vi "Prog Interface - TREE.vi"() -> ()   [LabVIEW 2017, in "Nanonis Prog Interface.lvlib"]
uses:
  Nanonis Prog Interface.lvlib
  <userlib>/Nanonis Prog Interface V5/Scan/Piezos/Piezo Calibration Sens Set.vi
  <userlib>/Nanonis Prog Interface V5/Scan/Piezos/Piezo Calibration Sens Get.vi
  <userlib>/Nanonis Prog Interface V5/Scan/Grid/GridPatternSet.vi
  <userlib>/Nanonis Prog Interface V5/Scan/Grid/GridPatternGet.vi
panel:
  in  "Tab Control":enum32{"Readme", "Version history"}(tab)=enum."Version history"
  in  "Version history":string="*** R8177 (September 2018) ***\n\nNew functions to get/set the limits of the User Outputs.\nNew functions to get values from the measurements list.\nAdapted function to get/set the properties of the Lockin Frequency Sweep.\n\n-----------------------------------------------------------------------------------------------------\n\n*** R8101 (September 2018) ***\n\nAdapted function to set the Idle value of the Fast Output from any connected SC5.\nAdapted function to get parameters from all modules to retrieve also the parameters grouped by module.\nAdapted function to get/set Scan properties to include the modules parameters selected in the Scan Control.\nNew function to open the Data Logger module.\nNew functions to get/set the XYZ voltage limits in the Piezo Calibration module.\nAdded option to wait until the tip stops withdrawing in the Withdraw function.\n\n-----------------------------------------------------------------------------------------------------\n\n*** R7861 (April 2018) ***\n\nNew functions palette for the Data Logger module.\n\n-----------------------------------------------------------------------------------------------------\n\n*** R7824 (April 2018) ***\n\nAdapted functions to the get/set the 2nd Auto Retract condition in the Z-Spectroscopy module.\n\n-----------------------------------------------------------------------------------------------------\n\n*** R7703 (February 2018) ***\n\nAdapted functions to the new number of available Real Time signals in the Nanonis software. \nThe full list of signals has increased from 80 to 128.\n\nAdded settling time to get/set properties of the Generic sweeper.\nAdded new functions to get/set Bias Spectroscopy options in the Advanced section.\nAdded optimizations to the get/set pattern functions when doing experiments on a grid.\n\n-----------------------------------------------------------------------------------------------------\n\n*** R7296 (June 2017) ***\n\nAdded functions to load/save LUTs in the Script-LUT Editor.\nIncreased the maximum number of steps allowed in the Generic Sweeper.\nAdded example to convert black pixels of an image into scan coordinates.\n\n-----------------------------------------------------------------------------------------------------\n\n*** R6949 (November 2016) ***\n\nAdded functions to get/set the configuration options in the Oscilation Control Signal Analyzer and Zoom FFT modules.\nDocumentation fix for Generic PI Controller.\n\n-----------------------------------------------------------------------------------------------------\n\n*** R6864 (October 2016) ***\n\nAdded a new function to set the Session folder.\n\n-----------------------------------------------------------------------------------------------------\n\n*** R6828 (September 2016) ***\n\nAdded new functions for the Function Generator (2 Channels) module.\nAdded new functions to Get / Set name and SI units of USer Outputs and User Inputs.\nAdded some VIs to the \"TREE.vi\" which were previously missing.\n\n-----------------------------------------------------------------------------------------------------\n\n*** R6778 (August 2016) ***\n\nAdded new functions for Modulator and demodulator channel set and get for Lockin, moved old VIs to Legacy (Removed from palettes).\nAdded Generic PI functions to set input and output channels.\n\n-----------------------------------------------------------------------------------------------------\n\n*** R6727 (August 2016) ***\n\nAdaptation to software with 80 channels and support for up to 3 SC5s, providing up to 16 additional outputs and 16 additional input channels.\n\n-----------------------------------------------------------------------------------------------------\n\n*** R6313 (March 2016) ***\n\nAdded Modulator phase offset to Lockin API\n\n-----------------------------------------------------------------------------------------------------\n\n*** R6310 (February 2016) ***\n\nNew functions to control the new Lock-in module. The old functions are still available as legacy VIs, but we strongly recommend using the new function set.\nNew functions for the Script module.\nNew example: History Chart 1-Channel (similar to the software built-in History graph)\n\n-----------------------------------------------------------------------------------------------------\n\n*** R6213 (January 2016) ***\n\nSome functions fixed.\n\n-----------------------------------------------------------------------------------------------------\n\n*** R6104 (November 2015) ***\n\nNew functions to load/save layouts, and to show/hide the PSD section of the High Resolution Oscilloscope.\n\n-----------------------------------------------------------------------------------------------------\n\n*** R5929 (October 2015) ***\n\nNew functions to draw multiple points and lines in the scan display.\n\n-----------------------------------------------------------------------------------------------------\n\n*** R5882 (September 2015) ***\n\nNew functions to get/set the Trigger Level value in the Oscilloscope High Resolution graph.\n\n-----------------------------------------------------------------------------------------------------\n\n*** R5864 (September 2015) ***\n\nNew functions to get/set the Withdraw Slew Rate in Z-Controller.\n\n-----------------------------------------------------------------------------------------------------\n\n*** R5786 (August 2015) ***\n\nNew functions to load/save settings files.\n\n-----------------------------------------------------------------------------------------------------\n\n*** R5706 (July 2015) ***\n\nThe examples are no longer part of the Nanonis library.\n\n-----------------------------------------------------------------------------------------------------\n\n*** R5681 (July 2015) ***\n\nNew function to open the Oscilloscope High Resolution graph.\n\n-----------------------------------------------------------------------------------------------------\n\n*** R5638 (June 2015) ***\n\nNew functions to control the Oscilloscope High Resolution graph.\nNew arrangement of functions inside subpalettes  in the Graphs palette.\nAdded more properties to the Properties Get/Set functions for Bias and Z spectroscopies.\n\n-----------------------------------------------------------------------------------------------------\n\n\n*** R5526 (April 2015) ***\n\nNew function to determine the optimal PLL gains.\n\n-----------------------------------------------------------------------------------------------------\n\n*** R5443 (March 2015) ***\n\nMultipass Callback VI example added a new input called \"Method\" to the connector pane. Now the Multipass example allows to execute user-defined code before (\"init\"), during (\"run\"), and after (\"end\") the scan.\n\n-----------------------------------------------------------------------------------------------------\n\n*** R5350 (February 2015) ***\n\nNew VIs in the Z-Controller palette to enable, get and set the Z limits.\n\n-----------------------------------------------------------------------------------------------------\n\n*** V5 first release R5286 (February 2015) ***\n\n-----------------------------------------------------------------------------------------------------\n\n*** R4760 (September 2014) ***\n\nNew VIs in the Current palette to get and set the calibration and offset.\n\n-----------------------------------------------------------------------------------------------------\n\n*** R4695 (June 2014) ***\n\nNew VIs in the Generic Sweeper palette to get properties and limits, and to stop the sweep.\n\n-----------------------------------------------------------------------------------------------------\n\n*** R4647 (May 2014) ***\n\nNew VIs to access the Global Counter.\n\n-----------------------------------------------------------------------------------------------------\n\n*** R4602 (April 2014) ***\n\nChanged VI:\n- HVA Info Get: added AUX gain.\n\n\n-----------------------------------------------------------------------------------------------------\n\n*** R4540 (February 2014) ***\n\nNew VIs:\n- Oscillation Control /-2 Lock-in Harmonic get / set\n- PLL Signal Analyzer and ZoomFFT: Open module, Channels get / set\n\nChanged VI:\n- Scan Speed Get / Set: added Bwd-Fwd Speed Ratio.\n\n\n-----------------------------------------------------------------------------------------------------\n\n*** R4316 (November 2013) ***\nNanonis Programming Interface V4.5 built by the VI Package Manager for the first time\n\n\n-----------------------------------------------------------------------------------------------------\n\n*** R4234 (October 2013) ***\n- New VIs to get/set the Beam Deflection configuration, in the Laser palette\n- New VIs to get/set the signals configuration in the Signals Manager, in the Signals palette\n\n\n-----------------------------------------------------------------------------------------------------\n\n*** V4.5 first release R3807 (May 2013) ***\nBased on Programming Interface V4.0, but including some changes:\n- Signal VIs adapted to the 48 signals available in V4.5\n- Support for new V4.5 Lock-in (FPGA Lock-in) and Oscilloscope 2T\n- New VIs to get/set the Function Generator idle value\n- Some other changes due to V4.5 modifications in the software"
  # "Programming Interface V5"
  # "See block diagram for VI TREE"
  # "1) What is the Programming Interface?\n\nThe Programming Interface is a set of LabVIEW VIs to control many functions of the Nanonis Controller Software.\n\n2) Location\n\nThe files are installed by default in the \"user.lib\" folder of LabVIEW.\nThus, the Programming Interface VIs are directly available from the LabVIEW function palette under the \"User libraries\" section. \nThe \"TREE.vi\" VI is not meant to be run but to display all the available VIs. \n\n3) Remote access\n\nIf you want to use the Programming Interface from another PC than the one on which the Nanonis Controller Software is running, you first have to enable the access from the Nanonis Software. \nTo do so, from the Nanonis Software main window, open the \"System>Options\" window and nagivate to \"Programming Interface\".\nIn the \"Machine access configuration\", add the IP address of the PC on which the Programming Interface VIs are running.\nMake sure your software firewall allows access from the remote PC. Depending on your software firewall you can add the remote PC in trusted environment or you can allow \"Nanonis SPM Controller.exe\" to listen to incoming connections and add port 3364 to the exceptions list.\n\n4) Examples\n\nSeveral example VIs are located in the \"Nanonis Prog Interface/Examples\" palette section."
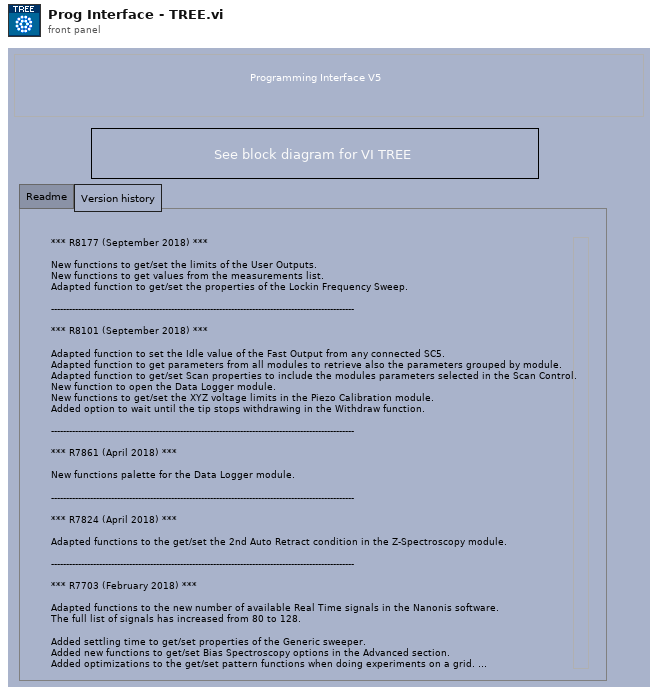
[diagram p1: front panel]
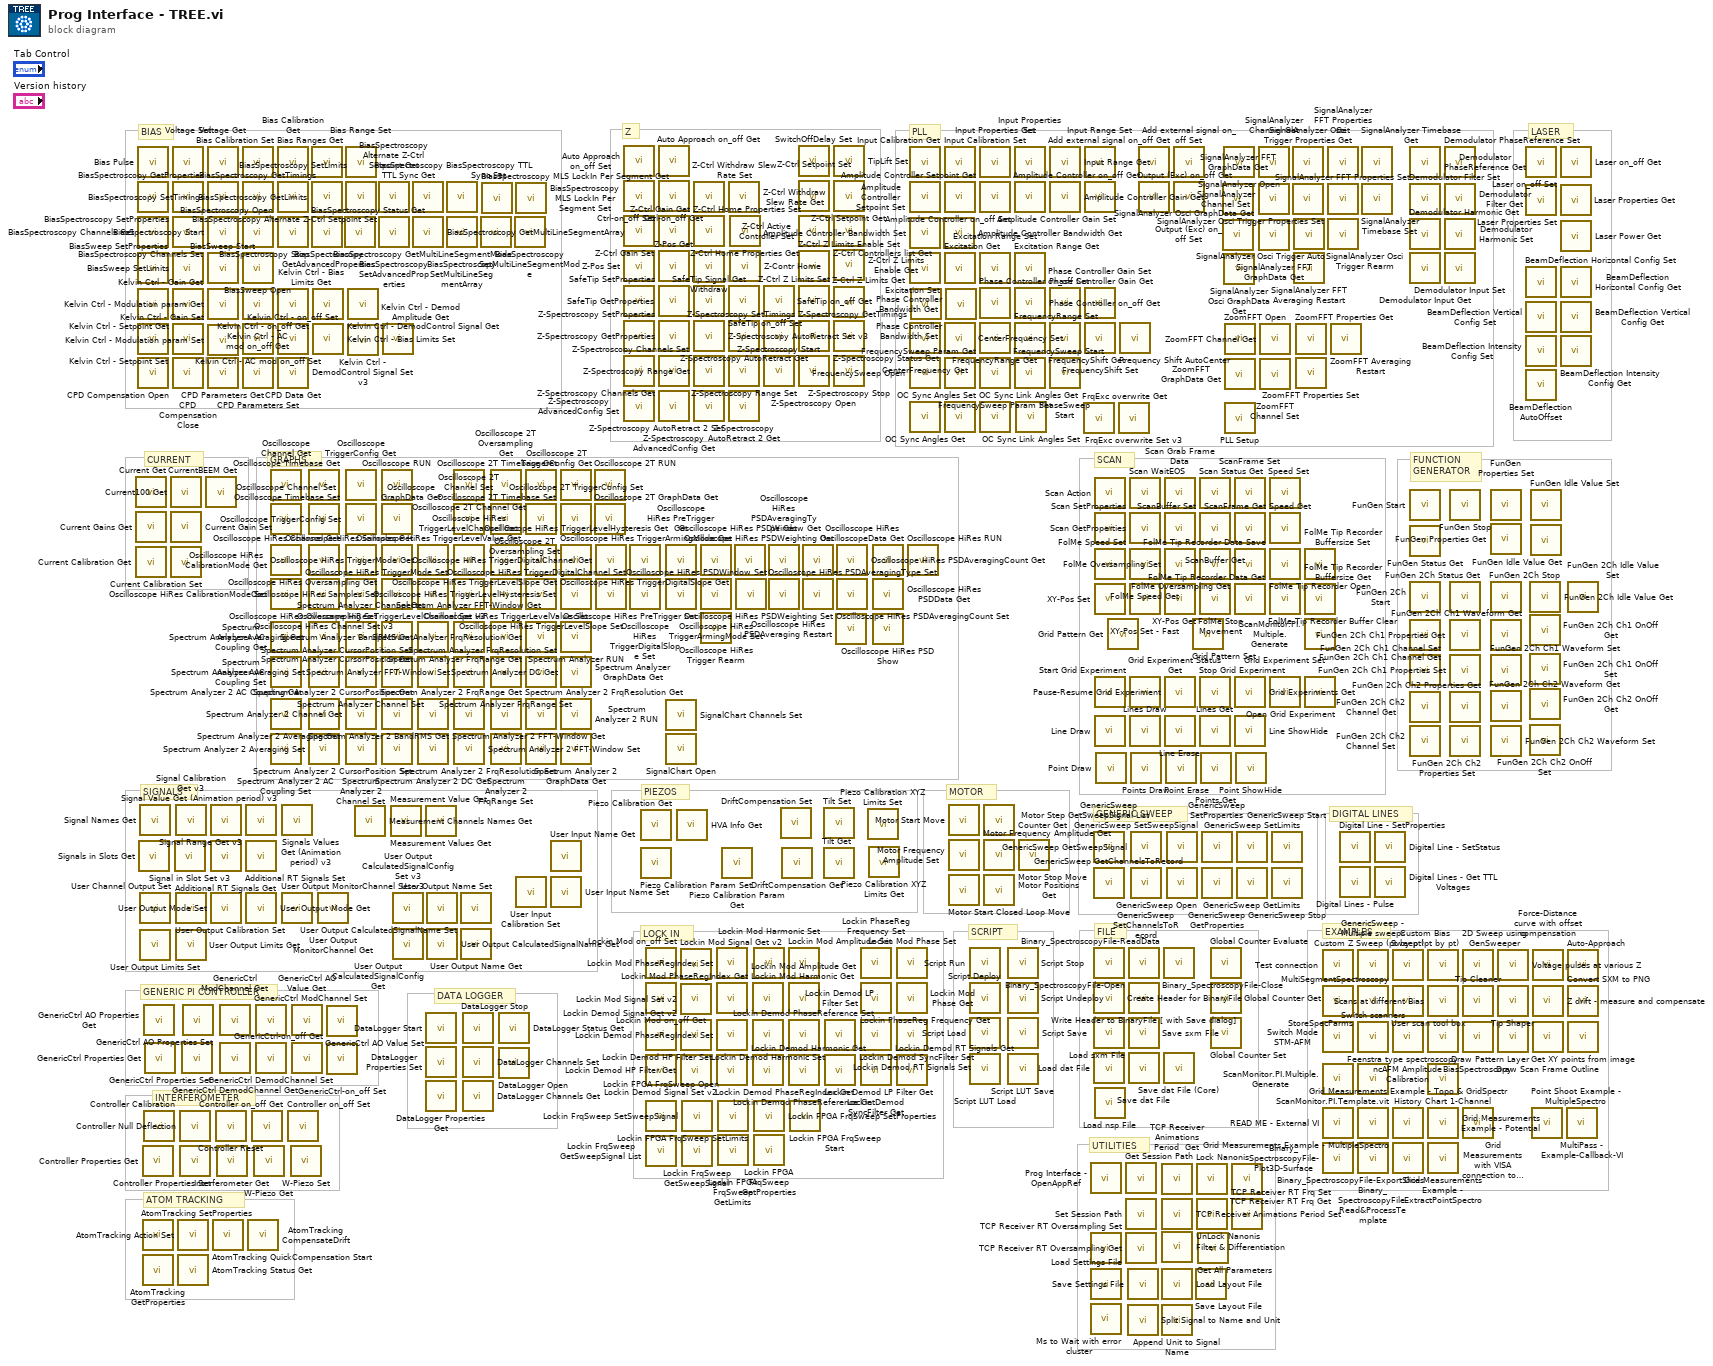
[diagram p0: block diagram]
diagram:
  # "DATA LOGGER"
  # "SCRIPT"
  # "LOCK IN"
  # "FUNCTION\nGENERATOR"
  # "GENERIC PI CONTROLLER"
  # "INTERFEROMETER"
  # "GRAPHS"
  # "LASER"
  # "ATOM TRACKING"
  # "PIEZOS"
  # "DIGITAL LINES"
  # "FILE"
  # "Z"
  # "UTILITIES"
  # "GENERIC SWEEP"
  # "SIGNALS"
  # "SCAN"
  # "PLL"
  # "EXAMPLES"
  # "CURRENT"
  # "MOTOR"
  # "BIAS"
  n1 = call <userlib>:"Current Get.vi"() -> ()  [unwired: 7 in, 3 out]
  n2 = call <userlib>:"Current Gains Get.vi"() -> ()  [unwired: 8 in, 4 out]
  n3 = call <userlib>:"Current Calibration Get.vi"() -> ()  [unwired: 8 in, 4 out]
  n4 = call <userlib>:"Bias Pulse.vi"() -> ()  [unwired: 14 in, 2 out]
  n5 = call <userlib>:"BiasSpectroscopy SetProperties.vi"() -> ()  [unwired: 14 in, 2 out]
  n6 = call <userlib>:"BiasSpectroscopy Channels Get.vi"() -> ()  [unwired: 9 in, 3 out]
  n7 = call <userlib>:"BiasSweep SetProperties.vi"() -> ()  [unwired: 14 in, 2 out]
  n8 = call <userlib>:"Kelvin Ctrl - Setpoint Get.vi"() -> ()  [unwired: 9 in, 3 out]
  n9 = call <userlib>:"Kelvin Ctrl - Setpoint Set.vi"() -> ()  [unwired: 10 in, 2 out]
  n10 = call <userlib>:"CPD Compensation Open.vi"() -> ()  [unwired: 14 in, 2 out]
  n11 = call <userlib>:"Signals in Slots Get.vi"() -> ()  [unwired: 6 in, 4 out]
  n12 = call <instrlib>:"Signal Names Get.vi"() -> ()  [unwired: 7 in, 3 out]
  n13 = call <userlib>:"User Channel Output Set.vi"() -> ()  [unwired: 9 in, 2 out]
  n14 = call <userlib>:"User Output Limits Set.vi"() -> ()  [unwired: 14 in, 2 out]
  n15 = call <userlib>:"Controller Properties Get.vi"() -> ()  [unwired: 11 in, 5 out]
  n16 = call <userlib>:"AtomTracking SetProperties.vi"() -> ()  [unwired: 14 in, 2 out]
  n17 = call <userlib>:"AtomTracking GetProperties.vi"() -> ()  [unwired: 9 in, 7 out]
  n18 = call <userlib>:"GenericCtrl AO Properties Get.vi"() -> ()  [unwired: 4 in, 8 out]
  n19 = call <userlib>:"Controller Calibration.vi"() -> ()  [unwired: 10 in, 2 out]
  n20 = call <userlib>:"GenericCtrl Properties Get.vi"() -> ()  [unwired: 6 in, 6 out]
  n21 = call <userlib>:"Current100 Get.vi"() -> ()  [unwired: 7 in, 3 out]
  n22 = call <userlib>:"Current Gain Set.vi"() -> ()  [unwired: 10 in, 2 out]
  n23 = call <userlib>:"Current Calibration Set.vi"() -> ()  [unwired: 10 in, 2 out]
  n24 = call <userlib>:"Voltage Set.vi"() -> ()  [unwired: 10 in, 2 out]
  n25 = call <userlib>:"BiasSpectroscopy GetProperties.vi"() -> ()  [unwired: 8 in, 8 out]
  n26 = call <userlib>:"BiasSpectroscopy Channels Set.vi"() -> ()  [unwired: 10 in, 2 out]
  n27 = call <userlib>:"BiasSweep SetLimits.vi"() -> ()  [unwired: 8 in, 2 out]
  n28 = call <userlib>:"Kelvin Ctrl - Gain Get.vi"() -> ()  [unwired: 11 in, 5 out]
  n29 = call <userlib>:"Kelvin Ctrl - Gain Set.vi"() -> ()  [unwired: 14 in, 2 out]
  n30 = call <userlib>:"CPD Compensation Close.vi"() -> ()  [unwired: 14 in, 2 out]
  n31 = call <userlib>:"Signal in Slot Set v3.vi"() -> ()  [unwired: 8 in, 2 out]
  n32 = call <userlib>:"Signal Calibration Get v3.vi"() -> ()  [unwired: 7 in, 4 out]
  n33 = call <userlib>:"User Output Calibration Set.vi"() -> ()  [unwired: 14 in, 2 out]
  n34 = call <userlib>:"User Output Limits Get.vi"() -> ()  [unwired: 12 in, 4 out]
  n35 = call <userlib>:"AtomTracking Action Set.vi"() -> ()  [unwired: 10 in, 2 out]
  n36 = call <userlib>:"AtomTracking Status Get.vi"() -> ()  [unwired: 9 in, 3 out]
  n37 = call <userlib>:"Controller Null Deflection.vi"() -> ()  [unwired: 10 in, 2 out]
  n38 = call <userlib>:"Controller Properties Set.vi"() -> ()  [unwired: 14 in, 2 out]
  n39 = call <userlib>:"GenericCtrl Properties Set.vi"() -> ()  [unwired: 10 in, 2 out]
  n40 = call <userlib>:"GenericCtrl AO Properties Set.vi"() -> ()  [unwired: 10 in, 2 out]
  n41 = call <userlib>:"CurrentBEEM Get.vi"() -> ()  [unwired: 7 in, 3 out]
  n42 = call <userlib>:"Voltage Get.vi"() -> ()  [unwired: 9 in, 3 out]
  n43 = call <userlib>:"BiasSpectroscopy SetTimings.vi"() -> ()  [unwired: 14 in, 2 out]
  n44 = call <userlib>:"BiasSpectroscopy Start.vi"() -> ()  [unwired: 11 in, 5 out]
  n45 = call <userlib>:"BiasSweep Start.vi"() -> ()  [unwired: 8 in, 4 out]
  n46 = call <userlib>:"Kelvin Ctrl - Modulation param Get.vi"() -> ()  [unwired: 11 in, 5 out]
  n47 = call <userlib>:"Kelvin Ctrl - Modulation param Set.vi"() -> ()  [unwired: 14 in, 2 out]
  n48 = call <userlib>:"CPD Parameters Get.vi"() -> ()  [unwired: 11 in, 5 out]
  n49 = call <userlib>:"Signal Range Get v3.vi"() -> ()  [unwired: 7 in, 4 out]
  n50 = call <userlib>:"Additional RT Signals Get.vi"() -> ()  [unwired: 11 in, 5 out]
  n51 = call <userlib>:"User Output Mode Set.vi"() -> ()  [unwired: 9 in, 2 out]
  n52 = call <userlib>:"AtomTracking QuickCompensation Start.vi"() -> ()  [unwired: 10 in, 2 out]
  n53 = call <userlib>:"Controller Reset.vi"() -> ()  [unwired: 10 in, 2 out]
  n54 = call <userlib>:"Interferometer Get.vi"() -> ()  [unwired: 9 in, 3 out]
  n55 = call <userlib>:"GenericCtrl ModChannel Get.vi"() -> ()  [unwired: 9 in, 3 out]
  n56 = call <userlib>:"GenericCtrl DemodChannel Get.vi"() -> ()  [unwired: 9 in, 3 out]
  n57 = call <userlib>:"Bias Calibration Set.vi"() -> ()  [unwired: 10 in, 2 out]
  n58 = call <userlib>:"BiasSpectroscopy GetTimings.vi"() -> ()  [unwired: 11 in, 5 out]
  n59 = call <userlib>:"BiasSpectroscopy Open.vi"() -> ()  [unwired: 14 in, 2 out]
  n60 = call <userlib>:"BiasSweep Open.vi"() -> ()  [unwired: 14 in, 2 out]
  n61 = call <userlib>:"Kelvin Ctrl - AC mod on_off Get.vi"() -> ()  [unwired: 8 in, 4 out]
  n62 = call <userlib>:"Kelvin Ctrl - AC mod on_off Set.vi"() -> ()  [unwired: 10 in, 2 out]
  n63 = call <userlib>:"CPD Parameters Set.vi"() -> ()  [unwired: 14 in, 2 out]
  n64 = call <instrlib>:"Signal Value Get (Animation period) v3.vi"() -> ()  [unwired: 8 in, 3 out]
  n65 = call <userlib>:"Additional RT Signals Set.vi"() -> ()  [unwired: 8 in, 2 out]
  n66 = call <userlib>:"User Output Mode Get.vi"() -> ()  [unwired: 7 in, 3 out]
  n67 = call <userlib>:"AtomTracking CompensateDrift.vi"() -> ()  [unwired: 10 in, 2 out]
  n68 = call <userlib>:"Controller on_off Get.vi"() -> ()  [unwired: 9 in, 3 out]
  n69 = call <userlib>:"W-Piezo Get.vi"() -> ()  [unwired: 9 in, 3 out]
  n70 = call <userlib>:"GenericCtrl ModChannel Set.vi"() -> ()  [unwired: 10 in, 2 out]
  n71 = call <userlib>:"GenericCtrl DemodChannel Set.vi"() -> ()  [unwired: 10 in, 2 out]
  n72 = call <userlib>:"Oscilloscope Channel Get.vi"() -> ()  [unwired: 9 in, 3 out]
  n73 = call <userlib>:"Oscilloscope Channel Set.vi"() -> ()  [unwired: 10 in, 2 out]
  n74 = call <userlib>:"Oscilloscope HiRes CalibrationMode Get.vi"() -> ()  [unwired: 9 in, 3 out]
  n75 = call <userlib>:"Oscilloscope HiRes CalibrationMode Set.vi"() -> ()  [unwired: 10 in, 2 out]
  n76 = call <userlib>:"Spectrum Analyzer AC Coupling Get.vi"() -> ()  [unwired: 9 in, 3 out]
  n77 = call <userlib>:"Spectrum Analyzer AC Coupling Set.vi"() -> ()  [unwired: 10 in, 2 out]
  n78 = call <userlib>:"Spectrum Analyzer 2 AC Coupling Get.vi"() -> ()  [unwired: 9 in, 3 out]
  n79 = call <userlib>:"Spectrum Analyzer 2 AC Coupling Set.vi"() -> ()  [unwired: 10 in, 2 out]
  n80 = call <userlib>:"Bias Calibration Get.vi"() -> ()  [unwired: 8 in, 4 out]
  n81 = call <userlib>:"BiasSpectroscopy SetLimits.vi"() -> ()  [unwired: 8 in, 2 out]
  n82 = call <userlib>:"BiasSpectroscopy Stop.vi"() -> ()  [unwired: 14 in, 2 out]
  n83 = call <userlib>:"Kelvin Ctrl - on_off Get.vi"() -> ()  [unwired: 9 in, 3 out]
  n84 = call <userlib>:"Kelvin Ctrl - on_off Set.vi"() -> ()  [unwired: 10 in, 2 out]
  n85 = call <userlib>:"CPD Data Get.vi"() -> ()  [unwired: 11 in, 5 out]
  n86 = call <userlib>:"Signals Values Get (Animation period) v3.vi"() -> ()  [unwired: 8 in, 3 out]
  n87 = call <userlib>:"User Output MonitorChannel Set v3.vi"() -> ()  [unwired: 9 in, 2 out]
  n88 = call <userlib>:"Controller on_off Set.vi"() -> ()  [unwired: 10 in, 2 out]
  n89 = call <userlib>:"W-Piezo Set.vi"() -> ()  [unwired: 10 in, 2 out]
  n90 = call <userlib>:"GenericCtrl AO Value Get.vi"() -> ()  [unwired: 9 in, 3 out]
  n91 = call <userlib>:"GenericCtrl-on_off Get.vi"() -> ()  [unwired: 9 in, 3 out]
  n92 = call <userlib>:"Oscilloscope Timebase Get.vi"() -> ()  [unwired: 8 in, 4 out]
  n93 = call <userlib>:"Oscilloscope Timebase Set.vi"() -> ()  [unwired: 10 in, 2 out]
  n94 = call <userlib>:"Oscilloscope HiRes Channel Get.vi"() -> ()  [unwired: 9 in, 3 out]
  n95 = call <userlib>:"Oscilloscope HiRes Channel Set v3.vi"() -> ()  [unwired: 10 in, 2 out]
  n96 = call <userlib>:"Spectrum Analyzer Averaging Get.vi"() -> ()  [unwired: 9 in, 3 out]
  n97 = call <userlib>:"Spectrum Analyzer Averaging Set.vi"() -> ()  [unwired: 10 in, 2 out]
  n98 = call <userlib>:"Spectrum Analyzer 2 Averaging Get.vi"() -> ()  [unwired: 9 in, 3 out]
  n99 = call <userlib>:"Spectrum Analyzer 2 Averaging Set.vi"() -> ()  [unwired: 10 in, 2 out]
  n100 = call <userlib>:"Bias Ranges Get.vi"() -> ()  [unwired: 8 in, 4 out]
  n101 = call <userlib>:"BiasSpectroscopy GetLimits.vi"() -> ()  [unwired: 6 in, 4 out]
  n102 = call <userlib>:"BiasSpectroscopy Status Get.vi"() -> ()  [unwired: 7 in, 3 out]
  n103 = call <userlib>:"Kelvin Ctrl - Bias Limits Get.vi"() -> ()  [unwired: 8 in, 4 out]
  n104 = call <userlib>:"Kelvin Ctrl - Bias Limits Set.vi"() -> ()  [unwired: 10 in, 2 out]
  n105 = call <userlib>:"User Output MonitorChannel Get.vi"() -> ()  [unwired: 8 in, 3 out]
  n106 = call <userlib>:"GenericCtrl AO Value Set.vi"() -> ()  [unwired: 10 in, 2 out]
  n107 = call <userlib>:"GenericCtrl-on_off Set.vi"() -> ()  [unwired: 10 in, 2 out]
  n108 = call <userlib>:"BiasSpectroscopy GetAdvancedProperties.vi"() -> ()  [unwired: 10 in, 6 out]
  n109 = call <userlib>:"Bias Range Set.vi"() -> ()  [unwired: 10 in, 2 out]
  n110 = call <userlib>:"BiasSpectroscopy Alternate Z-Ctrl Setpoint Set.vi"() -> ()  [unwired: 14 in, 2 out]
  n111 = call <userlib>:"Oscilloscope TriggerConfig Get.vi"() -> ()  [unwired: 8 in, 4 out]
  n112 = call <userlib>:"Oscilloscope TriggerConfig Set.vi"() -> ()  [unwired: 10 in, 2 out]
  n113 = call <userlib>:"Oscilloscope HiRes Oversampling Get.vi"() -> ()  [unwired: 9 in, 3 out]
  n114 = call <userlib>:"Oscilloscope HiRes Oversampling Set.vi"() -> ()  [unwired: 10 in, 2 out]
  n115 = call <userlib>:"Spectrum Analyzer Channel Get.vi"() -> ()  [unwired: 9 in, 3 out]
  n116 = call <userlib>:"Spectrum Analyzer Channel Set.vi"() -> ()  [unwired: 10 in, 2 out]
  n117 = call <userlib>:"Spectrum Analyzer 2 Channel Get.vi"() -> ()  [unwired: 9 in, 3 out]
  n118 = call <userlib>:"Spectrum Analyzer 2 Channel Set.vi"() -> ()  [unwired: 10 in, 2 out]
  n119 = call <userlib>:"Kelvin Ctrl - DemodControl Signal Get.vi"() -> ()  [unwired: 9 in, 3 out]
  n120 = call <userlib>:"Kelvin Ctrl - DemodControl Signal Set v3.vi"() -> ()  [unwired: 10 in, 2 out]
  n121 = call <userlib>:"Measurement Channels Names Get.vi"() -> ()  [unwired: 9 in, 3 out]
  n122 = call <userlib>:"BiasSpectroscopy Alternate Z-Ctrl Setpoint Get.vi"() -> ()  [unwired: 11 in, 5 out]
  n123 = call <userlib>:"BiasSpectroscopy SetAdvancedProperties.vi"() -> ()  [unwired: 14 in, 2 out]
  n124 = call <userlib>:"Oscilloscope RUN.vi"() -> ()  [unwired: 10 in, 2 out]
  n125 = call <userlib>:"Oscilloscope GraphData Get.vi"() -> ()  [unwired: 9 in, 3 out]
  n126 = call <userlib>:"Oscilloscope HiRes Samples Get.vi"() -> ()  [unwired: 9 in, 3 out]
  n127 = call <userlib>:"Oscilloscope HiRes Samples Set.vi"() -> ()  [unwired: 10 in, 2 out]
  n128 = call <userlib>:"Spectrum Analyzer CursorPosition Get.vi"() -> ()  [unwired: 11 in, 5 out]
  n129 = call <userlib>:"Spectrum Analyzer CursorPosition Set.vi"() -> ()  [unwired: 14 in, 2 out]
  n130 = call <userlib>:"Spectrum Analyzer 2 CursorPosition Get.vi"() -> ()  [unwired: 11 in, 5 out]
  n131 = call <userlib>:"Spectrum Analyzer 2 CursorPosition Set.vi"() -> ()  [unwired: 14 in, 2 out]
  n132 = call <userlib>:"Kelvin Ctrl - Demod Amplitude Get.vi"() -> ()  [unwired: 9 in, 3 out]
  n133 = call <userlib>:"Measurement Value Get.vi"() -> ()  [unwired: 8 in, 3 out]
  n134 = call <userlib>:"User Output CalculatedSignalConfig Set v3.vi"() -> ()  [unwired: 9 in, 2 out]
  n135 = call <userlib>:"User Output CalculatedSignalConfig Get.vi"() -> ()  [unwired: 8 in, 3 out]
  n136 = call <userlib>:"BiasSpectroscopy TTL Sync Get.vi"() -> ()  [unwired: 9 in, 7 out]
  n137 = call <userlib>:"BiasSpectroscopy GetMultiLineSegmentArray.vi"() -> ()  [unwired: 7 in, 3 out]
  n138 = call <userlib>:"Oscilloscope HiRes TriggerMode Get.vi"() -> ()  [unwired: 9 in, 3 out]
  n139 = call <userlib>:"Oscilloscope HiRes TriggerMode Set.vi"() -> ()  [unwired: 10 in, 2 out]
  n140 = call <userlib>:"Spectrum Analyzer BandRMS Get.vi"() -> ()  [unwired: 8 in, 4 out]
  n141 = call <userlib>:"Spectrum Analyzer DC Get.vi"() -> ()  [unwired: 9 in, 3 out]
  n142 = call <userlib>:"Spectrum Analyzer 2 BandRMS Get.vi"() -> ()  [unwired: 8 in, 4 out]
  n143 = call <userlib>:"Spectrum Analyzer 2 DC Get.vi"() -> ()  [unwired: 9 in, 3 out]
  n144 = call <userlib>:"Measurement Values Get.vi"() -> ()  [unwired: 8 in, 3 out]
  n145 = call <userlib>:"DataLogger Start.vi"() -> ()  [unwired: 14 in, 2 out]
  n146 = call <userlib>:"DataLogger Properties Set.vi"() -> ()  [unwired: 10 in, 2 out]
  n147 = call <userlib>:"DataLogger Properties Get.vi"() -> ()  [unwired: 7 in, 5 out]
  n148 = call <userlib>:"User Output CalculatedSignalName Set.vi"() -> ()  [unwired: 9 in, 2 out]
  n149 = call <userlib>:"User Output CalculatedSignalName Get.vi"() -> ()  [unwired: 8 in, 3 out]
  n150 = call <userlib>:"BiasSpectroscopy TTL Sync Set.vi"() -> ()  [unwired: 14 in, 2 out]
  n151 = call <userlib>:"BiasSpectroscopy SetMultiLineSegmentArray.vi"() -> ()  [unwired: 8 in, 2 out]
  n152 = call <userlib>:"Oscilloscope 2T Channel Get.vi"() -> ()  [unwired: 8 in, 4 out]
  n153 = call <userlib>:"Oscilloscope 2T Channel Set.vi"() -> ()  [unwired: 10 in, 2 out]
  n154 = call <userlib>:"Oscilloscope HiRes TriggerLevelChannel Get.vi"() -> ()  [unwired: 9 in, 3 out]
  n155 = call <userlib>:"Oscilloscope HiRes TriggerLevelChannel Set v3.vi"() -> ()  [unwired: 10 in, 2 out]
  n156 = call <userlib>:"Spectrum Analyzer FFT-Window Get.vi"() -> ()  [unwired: 9 in, 3 out]
  n157 = call <userlib>:"Spectrum Analyzer FFT-Window Set.vi"() -> ()  [unwired: 10 in, 2 out]
  n158 = call <userlib>:"Spectrum Analyzer 2 FFT-Window Get.vi"() -> ()  [unwired: 9 in, 3 out]
  n159 = call <userlib>:"Spectrum Analyzer 2 FFT-Window Set.vi"() -> ()  [unwired: 10 in, 2 out]
  n160 = call <userlib>:"User Output Name Set.vi"() -> ()  [unwired: 14 in, 2 out]
  n161 = call <userlib>:"User Output Name Get.vi"() -> ()  [unwired: 12 in, 4 out]
  n162 = call <userlib>:"DataLogger Stop.vi"() -> ()  [unwired: 14 in, 2 out]
  n163 = call <userlib>:"DataLogger Channels Set.vi"() -> ()  [unwired: 10 in, 2 out]
  n164 = call <userlib>:"DataLogger Channels Get.vi"() -> ()  [unwired: 9 in, 3 out]
  n165 = call <userlib>:"BiasSpectroscopy GetMultiLineSegmentMode.vi"() -> ()  [unwired: 7 in, 3 out]
  n166 = call <userlib>:"BiasSpectroscopy MLS LockIn Per Segment Get.vi"() -> ()  [unwired: 9 in, 3 out]
  n167 = call <userlib>:"Oscilloscope 2T Oversampling Get.vi"() -> ()  [unwired: 8 in, 3 out]
  n168 = call <userlib>:"Oscilloscope 2T Oversampling Set.vi"() -> ()  [unwired: 10 in, 2 out]
  n169 = call <userlib>:"Oscilloscope HiRes TriggerLevelValue Get.vi"() -> ()  [unwired: 9 in, 3 out]
  n170 = call <userlib>:"Oscilloscope HiRes TriggerLevelValue Set.vi"() -> ()  [unwired: 10 in, 2 out]
  n171 = call <userlib>:"Spectrum Analyzer FrqRange Get.vi"() -> ()  [unwired: 8 in, 4 out]
  n172 = call <userlib>:"Spectrum Analyzer FrqRange Set.vi"() -> ()  [unwired: 10 in, 2 out]
  n173 = call <userlib>:"Spectrum Analyzer 2 FrqRange Get.vi"() -> ()  [unwired: 8 in, 4 out]
  n174 = call <userlib>:"Spectrum Analyzer 2 FrqRange Set.vi"() -> ()  [unwired: 10 in, 2 out]
  n175 = call <userlib>:"DataLogger Status Get.vi"() -> ()  [unwired: 7 in, 4 out]
  n176 = call <userlib>:"DataLogger Open.vi"() -> ()  [unwired: 14 in, 2 out]
  n177 = call <userlib>:"BiasSpectroscopy SetMultiLineSegmentMode.vi"() -> ()  [unwired: 8 in, 2 out]
  n178 = call <userlib>:"BiasSpectroscopy MLS LockIn Per Segment Set.vi"() -> ()  [unwired: 10 in, 2 out]
  n179 = call <userlib>:"User Input Calibration Set.vi"() -> ()  [unwired: 14 in, 2 out]
  n180 = call <userlib>:"Oscilloscope 2T Timebase Get.vi"() -> ()  [unwired: 8 in, 4 out]
  n181 = call <userlib>:"Oscilloscope 2T Timebase Set.vi"() -> ()  [unwired: 10 in, 2 out]
  n182 = call <userlib>:"Oscilloscope HiRes TriggerLevelSlope Get.vi"() -> ()  [unwired: 9 in, 3 out]
  n183 = call <userlib>:"Oscilloscope HiRes TriggerLevelSlope Set.vi"() -> ()  [unwired: 10 in, 2 out]
  n184 = call <userlib>:"Spectrum Analyzer FrqResolution Get.vi"() -> ()  [unwired: 8 in, 4 out]
  n185 = call <userlib>:"Spectrum Analyzer FrqResolution Set.vi"() -> ()  [unwired: 10 in, 2 out]
  n186 = call <userlib>:"Spectrum Analyzer 2 FrqResolution Get.vi"() -> ()  [unwired: 8 in, 4 out]
  n187 = call <userlib>:"Spectrum Analyzer 2 FrqResolution Set.vi"() -> ()  [unwired: 10 in, 2 out]
  n188 = call <userlib>:"User Input Name Get.vi"() -> ()  [unwired: 12 in, 4 out]
  n189 = call <userlib>:"User Input Name Set.vi"() -> ()  [unwired: 14 in, 2 out]
  n190 = call <userlib>:"Oscilloscope 2T TriggerConfig Get.vi"() -> ()  [unwired: 8 in, 4 out]
  n191 = call <userlib>:"Oscilloscope 2T TriggerConfig Set.vi"() -> ()  [unwired: 10 in, 2 out]
  n192 = call <userlib>:"Oscilloscope HiRes TriggerLevelHysteresis Get.vi"() -> ()  [unwired: 9 in, 3 out]
  n193 = call <userlib>:"Oscilloscope HiRes TriggerLevelHysteresis Set.vi"() -> ()  [unwired: 10 in, 2 out]
  n194 = call <userlib>:"Spectrum Analyzer RUN.vi"() -> ()  [unwired: 10 in, 2 out]
  n195 = call <userlib>:"Spectrum Analyzer GraphData Get.vi"() -> ()  [unwired: 9 in, 3 out]
  n196 = call <userlib>:"Spectrum Analyzer 2 RUN.vi"() -> ()  [unwired: 10 in, 2 out]
  n197 = call <userlib>:"Spectrum Analyzer 2 GraphData Get.vi"() -> ()  [unwired: 9 in, 3 out]
  n198 = call <userlib>:"Oscilloscope 2T RUN.vi"() -> ()  [unwired: 10 in, 2 out]
  n199 = call <userlib>:"Oscilloscope 2T GraphData Get.vi"() -> ()  [unwired: 9 in, 3 out]
  n200 = call <userlib>:"Oscilloscope HiRes TriggerDigitalChannel Get.vi"() -> ()  [unwired: 9 in, 3 out]
  n201 = call <userlib>:"Oscilloscope HiRes TriggerDigitalChannel Set.vi"() -> ()  [unwired: 10 in, 2 out]
  n202 = call <userlib>:"Auto Approach on_off Set.vi"() -> ()  [unwired: 8 in, 2 out]
  n203 = call <userlib>:"Ctrl-on_off Set.vi"() -> ()  [unwired: 10 in, 2 out]
  n204 = call <userlib>:"Z-Ctrl Gain Set.vi"() -> ()  [unwired: 9 in, 2 out]
  n205 = call <userlib>:"Z-Pos Set.vi"() -> ()  [unwired: 10 in, 2 out]
  n206 = call <userlib>:"SafeTip SetProperties.vi"() -> ()  [unwired: 14 in, 2 out]
  n207 = call <userlib>:"Z-Spectroscopy SetProperties.vi"() -> ()  [unwired: 14 in, 2 out]
  n208 = call <userlib>:"Z-Spectroscopy Channels Get.vi"() -> ()  [unwired: 9 in, 3 out]
  n209 = call <userlib>:"Z-Spectroscopy AdvancedConfig Set.vi"() -> ()  [unwired: 14 in, 2 out]
  n210 = call <userlib>:"Oscilloscope HiRes TriggerDigitalSlope Get.vi"() -> ()  [unwired: 9 in, 3 out]
  n211 = call <userlib>:"Oscilloscope HiRes TriggerDigitalSlope Set.vi"() -> ()  [unwired: 10 in, 2 out]
  n212 = call <userlib>:"Piezo Calibration Get.vi"() -> ()  [unwired: 11 in, 5 out]
  n213 = call-poly "Piezo Calibration Param Set.vi"() -> ()  [unwired: 14 in, 2 out]
  n214 = call <userlib>:"Lockin Mod on_off Set.vi"() -> ()  [unwired: 10 in, 2 out]
  n215 = call <userlib>:"Lockin Mod on_off Get.vi"() -> ()  [unwired: 9 in, 3 out]
  n216 = call <userlib>:"Lockin Demod Signal Get v2.vi"() -> ()  [unwired: 9 in, 3 out]
  n217 = call <userlib>:"Lockin Demod Signal Set v2.vi"() -> ()  [unwired: 10 in, 2 out]
  n218 = call <userlib>:"Lockin FPGA FrqSweep Open.vi"() -> ()  [unwired: 10 in, 2 out]
  n219 = call <userlib>:"Lockin FrqSweep GetSweepSignal List.vi"() -> ()  [unwired: 9 in, 3 out]
  n220 = call <userlib>:"Auto Approach on_off Get.vi"() -> ()  [unwired: 7 in, 3 out]
  n221 = call <userlib>:"Ctrl-on_off Get.vi"() -> ()  [unwired: 9 in, 3 out]
  n222 = call <userlib>:"Z-Ctrl Gain Get.vi"() -> ()  [unwired: 11 in, 5 out]
  n223 = call <userlib>:"Z-Pos Get.vi"() -> ()  [unwired: 9 in, 3 out]
  n224 = call <userlib>:"SafeTip GetProperties.vi"() -> ()  [unwired: 11 in, 5 out]
  n225 = call <userlib>:"Z-Spectroscopy GetProperties.vi"() -> ()  [unwired: 8 in, 8 out]
  n226 = call <userlib>:"Z-Spectroscopy Channels Set.vi"() -> ()  [unwired: 10 in, 2 out]
  n227 = call <userlib>:"Z-Spectroscopy AdvancedConfig Get.vi"() -> ()  [unwired: 10 in, 6 out]
  n228 = call <userlib>:"Oscilloscope HiRes PreTrigger Get.vi"() -> ()  [unwired: 9 in, 3 out]
  n229 = call <userlib>:"Oscilloscope HiRes PreTrigger Set.vi"() -> ()  [unwired: 10 in, 2 out]
  n230 = call <userlib>:"SignalChart Channels Set.vi"() -> ()  [unwired: 10 in, 2 out]
  n231 = call <userlib>:"SignalChart Open.vi"() -> ()  [unwired: 10 in, 2 out]
  n232 = call <userlib>:"HVA Info Get.vi"() -> ()  [unwired: 7 in, 5 out]
  n233 = call <userlib>:"Lockin Mod Signal Get v2.vi"() -> ()  [unwired: 9 in, 3 out]
  n234 = call <userlib>:"Lockin Mod Signal Set v2.vi"() -> ()  [unwired: 10 in, 2 out]
  n235 = call <userlib>:"Lockin Demod HP Filter Set.vi"() -> ()  [unwired: 10 in, 2 out]
  n236 = call <userlib>:"Lockin Demod HP Filter Get.vi"() -> ()  [unwired: 8 in, 4 out]
  n237 = call <userlib>:"Lockin FrqSweep SetSweepSignal.vi"() -> ()  [unwired: 10 in, 2 out]
  n238 = call <userlib>:"Lockin FrqSweep GetSweepSignal.vi"() -> ()  [unwired: 8 in, 4 out]
  n239 = call <userlib>:"Z-Ctrl Withdraw Slew Rate Set.vi"() -> ()  [unwired: 10 in, 2 out]
  n240 = call <userlib>:"Z-Ctrl Home Properties Set.vi"() -> ()  [unwired: 9 in, 2 out]
  n241 = call <userlib>:"Withdraw.vi"() -> ()  [unwired: 10 in, 2 out]
  n242 = call <userlib>:"SafeTip Signal Get.vi"() -> ()  [unwired: 9 in, 3 out]
  n243 = call <userlib>:"Z-Spectroscopy AutoRetract Set v3.vi"() -> ()  [unwired: 10 in, 2 out]
  n244 = call <userlib>:"Z-Spectroscopy Range Get.vi"() -> ()  [unwired: 7 in, 4 out]
  n245 = call <userlib>:"Z-Spectroscopy AutoRetract 2 Set.vi"() -> ()  [unwired: 10 in, 2 out]
  n246 = call <userlib>:"Oscilloscope HiRes TriggerArmingMode Get.vi"() -> ()  [unwired: 9 in, 3 out]
  n247 = call <userlib>:"Oscilloscope HiRes TriggerArmingMode Set.vi"() -> ()  [unwired: 10 in, 2 out]
  n248 = call <userlib>:"Oscilloscope HiRes Trigger Rearm.vi"() -> ()  [unwired: 10 in, 2 out]
  n249 = call <userlib>:"Lockin Mod PhaseRegIndex Set.vi"() -> ()  [unwired: 10 in, 2 out]
  n250 = call <userlib>:"Lockin Mod PhaseRegIndex Get.vi"() -> ()  [unwired: 9 in, 3 out]
  n251 = call <userlib>:"Lockin Demod PhaseRegIndex Set.vi"() -> ()  [unwired: 10 in, 2 out]
  n252 = call <userlib>:"Lockin Demod PhaseRegIndex Get.vi"() -> ()  [unwired: 9 in, 3 out]
  n253 = call <userlib>:"Lockin FPGA FrqSweep SetLimits.vi"() -> ()  [unwired: 10 in, 2 out]
  n254 = call <userlib>:"Lockin FPGA FrqSweep GetLimits.vi"() -> ()  [unwired: 8 in, 4 out]
  n255 = call-poly "Piezo Calibration Param Get.vi"() -> ()  [unwired: 11 in, 5 out]
  n256 = call <userlib>:"Z-Ctrl Withdraw Slew Rate Get.vi"() -> ()  [unwired: 9 in, 3 out]
  n257 = call <userlib>:"SafeTip on_off Set.vi"() -> ()  [unwired: 10 in, 2 out]
  n258 = call <userlib>:"Z-Spectroscopy AutoRetract Get.vi"() -> ()  [unwired: 6 in, 6 out]
  n259 = call <userlib>:"Z-Spectroscopy Range Set.vi"() -> ()  [unwired: 9 in, 2 out]
  n260 = call <userlib>:"Z-Spectroscopy AutoRetract 2 Get.vi"() -> ()  [unwired: 6 in, 6 out]
  n261 = call <userlib>:"Z-Ctrl Home Properties Get.vi"() -> ()  [unwired: 7 in, 4 out]
  n262 = call <userlib>:"Z-Contr Home.vi"() -> ()  [unwired: 10 in, 2 out]
  n263 = call <userlib>:"Oscilloscope HiRes PSDWindow Get.vi"() -> ()  [unwired: 9 in, 3 out]
  n264 = call <userlib>:"Oscilloscope HiRes PSDWindow Set.vi"() -> ()  [unwired: 10 in, 2 out]
  n265 = call <userlib>:"Lockin Mod Harmonic Get.vi"() -> ()  [unwired: 9 in, 3 out]
  n266 = call <userlib>:"Lockin Demod Harmonic Set.vi"() -> ()  [unwired: 10 in, 2 out]
  n267 = call <userlib>:"Lockin Demod Harmonic Get.vi"() -> ()  [unwired: 9 in, 3 out]
  n268 = call <userlib>:"Lockin Mod Harmonic Set.vi"() -> ()  [unwired: 10 in, 2 out]
  n269 = call <userlib>:"Lockin FPGA FrqSweep SetProperties.vi"() -> ()  [unwired: 14 in, 2 out]
  n270 = call <userlib>:"Lockin FPGA FrqSweep GetProperties.vi"() -> ()  [unwired: 10 in, 6 out]
  n271 = call <userlib>:"SafeTip on_off Get.vi"() -> ()  [unwired: 9 in, 3 out]
  n272 = call <userlib>:"Z-Spectroscopy SetTimings.vi"() -> ()  [unwired: 14 in, 2 out]
  n273 = call <userlib>:"Z-Spectroscopy Start.vi"() -> ()  [unwired: 11 in, 5 out]
  n274 = call <userlib>:"Oscilloscope HiRes PSDAveragingType Get.vi"() -> ()  [unwired: 9 in, 3 out]
  n275 = call <userlib>:"Oscilloscope HiRes PSDAveragingType Set.vi"() -> ()  [unwired: 10 in, 2 out]
  n276 = call <userlib>:"DriftCompensation Set.vi"() -> ()  [unwired: 14 in, 2 out]
  n277 = call <userlib>:"DriftCompensation Get.vi"() -> ()  [unwired: 11 in, 5 out]
  n278 = call <userlib>:"Lockin Mod Amplitude Set.vi"() -> ()  [unwired: 10 in, 2 out]
  n279 = call <userlib>:"Lockin Mod Amplitude Get.vi"() -> ()  [unwired: 9 in, 3 out]
  n280 = call <userlib>:"Lockin Demod PhaseReference Set.vi"() -> ()  [unwired: 10 in, 2 out]
  n281 = call <userlib>:"Lockin Demod PhaseReference Get.vi"() -> ()  [unwired: 9 in, 3 out]
  n282 = call <userlib>:"Lockin FPGA FrqSweep Start.vi"() -> ()  [unwired: 8 in, 4 out]
  n283 = call <userlib>:"SwitchOffDelay Set.vi"() -> ()  [unwired: 10 in, 2 out]
  n284 = call <userlib>:"Z-Ctrl Setpoint Set.vi"() -> ()  [unwired: 10 in, 2 out]
  n285 = call <userlib>:"Z-Ctrl Active Controller Set.vi"() -> ()  [unwired: 10 in, 2 out]
  n286 = call <userlib>:"Z-Ctrl Z Limits Enable Set.vi"() -> ()  [unwired: 10 in, 2 out]
  n287 = call <userlib>:"Z-Ctrl Z Limits Set.vi"() -> ()  [unwired: 10 in, 2 out]
  n288 = call <userlib>:"Z-Spectroscopy GetTimings.vi"() -> ()  [unwired: 11 in, 5 out]
  n289 = call <userlib>:"Z-Spectroscopy Open.vi"() -> ()  [unwired: 14 in, 2 out]
  n290 = call <userlib>:"Oscilloscope HiRes PSDWeighting Get.vi"() -> ()  [unwired: 9 in, 3 out]
  n291 = call <userlib>:"Oscilloscope HiRes PSDWeighting Set.vi"() -> ()  [unwired: 10 in, 2 out]
  n292 = call <userlib>:"Tilt Set.vi"() -> ()  [unwired: 10 in, 2 out]
  n293 = call <userlib>:"Tilt Get.vi"() -> ()  [unwired: 8 in, 4 out]
  n294 = call <userlib>:"Lockin Demod LP Filter Set.vi"() -> ()  [unwired: 10 in, 2 out]
  n295 = call <userlib>:"Lockin Demod LP Filter Get.vi"() -> ()  [unwired: 8 in, 4 out]
  n296 = call <userlib>:"TipLift Set.vi"() -> ()  [unwired: 10 in, 2 out]
  n297 = call <userlib>:"Z-Ctrl Setpoint Get.vi"() -> ()  [unwired: 8 in, 3 out]
  n298 = call <userlib>:"Z-Ctrl Controllers list Get.vi"() -> ()  [unwired: 8 in, 4 out]
  n299 = call <userlib>:"Z-Ctrl Z Limits Enable Get.vi"() -> ()  [unwired: 9 in, 3 out]
  n300 = call <userlib>:"Z-Ctrl Z Limits Get.vi"() -> ()  [unwired: 8 in, 4 out]
  n301 = call <userlib>:"Z-Spectroscopy Status Get.vi"() -> ()  [unwired: 7 in, 3 out]
  n302 = call <userlib>:"Z-Spectroscopy Stop.vi"() -> ()  [unwired: 14 in, 2 out]
  n303 = call <userlib>:"Oscilloscope HiRes PSDAveraging Restart.vi"() -> ()  [unwired: 10 in, 2 out]
  n304 = call <userlib>:"Oscilloscope HiRes PSDAveragingCount Get.vi"() -> ()  [unwired: 9 in, 3 out]
  n305 = call <userlib>:"Oscilloscope HiRes PSDAveragingCount Set.vi"() -> ()  [unwired: 10 in, 2 out]
  n306 = call <userlib>:"Lockin PhaseReg Frequency Set.vi"() -> ()  [unwired: 10 in, 2 out]
  n307 = call <userlib>:"Lockin PhaseReg Frequency Get.vi"() -> ()  [unwired: 9 in, 3 out]
  n308 = call <userlib>:"Lockin Demod SyncFilter Set.vi"() -> ()  [unwired: 10 in, 2 out]
  n309 = call <userlib>:"Lockin Demod SyncFilter Get.vi"() -> ()  [unwired: 9 in, 3 out]
  n310 = call <userlib>:"Piezo Calibration XYZ Limits Set.vi"() -> ()  [unwired: 14 in, 2 out]
  n311 = call <userlib>:"Piezo Calibration XYZ Limits Get.vi"() -> ()  [unwired: 10 in, 6 out]
  n312 = call <userlib>:"Oscilloscope HiRes OscilloscopeData Get.vi"() -> ()  [unwired: 8 in, 4 out]
  n313 = call <userlib>:"Oscilloscope HiRes PSDData Get.vi"() -> ()  [unwired: 8 in, 4 out]
  n314 = call <userlib>:"Oscilloscope HiRes PSD Show.vi"() -> ()  [unwired: 10 in, 2 out]
  n315 = call <userlib>:"Lockin Mod Phase Set.vi"() -> ()  [unwired: 10 in, 2 out]
  n316 = call <userlib>:"Lockin Mod Phase Get.vi"() -> ()  [unwired: 9 in, 3 out]
  n317 = call <userlib>:"Lockin Demod RT Signals Set.vi"() -> ()  [unwired: 10 in, 2 out]
  n318 = call <userlib>:"Lockin Demod RT Signals Get.vi"() -> ()  [unwired: 9 in, 3 out]
  n319 = call <userlib>:"Oscilloscope HiRes RUN.vi"() -> ()  [unwired: 10 in, 2 out]
  n320 = call <userlib>:"Input Calibration Get.vi"() -> ()  [unwired: 9 in, 3 out]
  n321 = call <userlib>:"Amplitude Controller Setpoint Set.vi"() -> ()  [unwired: 10 in, 2 out]
  n322 = call <userlib>:"Amplitude Controller Bandwidth Set.vi"() -> ()  [unwired: 10 in, 2 out]
  n323 = call <userlib>:"Excitation Set.vi"() -> ()  [unwired: 10 in, 2 out]
  n324 = call <userlib>:"CenterFrequency Get.vi"() -> ()  [unwired: 9 in, 3 out]
  n325 = call <userlib>:"FrequencySweep Open.vi"() -> ()  [unwired: 10 in, 2 out]
  n326 = call <userlib>:"OC Sync Angles Get.vi"() -> ()  [unwired: 6 in, 4 out]
  n327 = call <userlib>:"Phase Controller Bandwidth Set.vi"() -> ()  [unwired: 10 in, 2 out]
  n328 = call <userlib>:"Amplitude Controller Bandwidth Get.vi"() -> ()  [unwired: 9 in, 3 out]
  n329 = call <userlib>:"Input Calibration Set.vi"() -> ()  [unwired: 10 in, 2 out]
  n330 = call <userlib>:"Amplitude Controller Setpoint Get.vi"() -> ()  [unwired: 9 in, 3 out]
  n331 = call <userlib>:"Excitation Get.vi"() -> ()  [unwired: 9 in, 3 out]
  n332 = call <userlib>:"CenterFrequency Set.vi"() -> ()  [unwired: 10 in, 2 out]
  n333 = call <userlib>:"FrequencySweep Param Get.vi"() -> ()  [unwired: 7 in, 5 out]
  n334 = call <userlib>:"OC Sync Angles Set.vi"() -> ()  [unwired: 8 in, 2 out]
  n335 = call <userlib>:"Phase Controller Bandwidth Get.vi"() -> ()  [unwired: 9 in, 3 out]
  n336 = call <userlib>:"Motor Start Move.vi"() -> ()  [unwired: 9 in, 2 out]
  n337 = call <userlib>:"Motor Frequency Amplitude Set.vi"() -> ()  [unwired: 10 in, 2 out]
  n338 = call <userlib>:"Motor Start Closed Loop Move.vi"() -> ()  [unwired: 14 in, 2 out]
  n339 = call <userlib>:"Script Run.vi"() -> ()  [unwired: 14 in, 2 out]
  n340 = call <userlib>:"Script Deploy.vi"() -> ()  [unwired: 14 in, 2 out]
  n341 = call <userlib>:"Script Load.vi"() -> ()  [unwired: 10 in, 2 out]
  n342 = call <userlib>:"Script LUT Load.vi"() -> ()  [unwired: 14 in, 2 out]
  n343 = call <userlib>:"Input Properties Get.vi"() -> ()  [unwired: 8 in, 4 out]
  n344 = call <userlib>:"Amplitude Controller on_off Set.vi"() -> ()  [unwired: 10 in, 2 out]
  n345 = call <userlib>:"Excitation Range Set.vi"() -> ()  [unwired: 10 in, 2 out]
  n346 = call <userlib>:"Phase Controller on_off Set.vi"() -> ()  [unwired: 10 in, 2 out]
  n347 = call <userlib>:"FrequencyRange Get.vi"() -> ()  [unwired: 9 in, 3 out]
  n348 = call <userlib>:"FrequencySweep Param Set.vi"() -> ()  [unwired: 10 in, 2 out]
  n349 = call <userlib>:"OC Sync Link Angles Get.vi"() -> ()  [unwired: 6 in, 4 out]
  n350 = call <userlib>:"Motor Step Counter Get.vi"() -> ()  [unwired: 11 in, 5 out]
  n351 = call <userlib>:"Motor Frequency Amplitude Get.vi"() -> ()  [unwired: 8 in, 4 out]
  n352 = call <userlib>:"Motor Positions Get.vi"() -> ()  [unwired: 11 in, 5 out]
  n353 = call <userlib>:"Script Stop.vi"() -> ()  [unwired: 14 in, 2 out]
  n354 = call <userlib>:"Script Undeploy.vi"() -> ()  [unwired: 14 in, 2 out]
  n355 = call <userlib>:"Script Save.vi"() -> ()  [unwired: 10 in, 2 out]
  n356 = call <userlib>:"Script LUT Save.vi"() -> ()  [unwired: 14 in, 2 out]
  n357 = call <userlib>:"Input Properties Set.vi"() -> ()  [unwired: 10 in, 2 out]
  n358 = call <userlib>:"Amplitude Controller on_off Get.vi"() -> ()  [unwired: 9 in, 3 out]
  n359 = call <userlib>:"Excitation Range Get.vi"() -> ()  [unwired: 9 in, 3 out]
  n360 = call <userlib>:"Phase Controller on_off Get.vi"() -> ()  [unwired: 9 in, 3 out]
  n361 = call <userlib>:"FrequencyRange Set.vi"() -> ()  [unwired: 10 in, 2 out]
  n362 = call <userlib>:"FrequencySweep Start.vi"() -> ()  [unwired: 7 in, 5 out]
  n363 = call <userlib>:"OC Sync Link Angles Set.vi"() -> ()  [unwired: 8 in, 2 out]
  n364 = call <userlib>:"Motor Stop Move.vi"() -> ()  [unwired: 10 in, 2 out]
  n365 = call <userlib>:"Input Range Get.vi"() -> ()  [unwired: 9 in, 3 out]
  n366 = call <userlib>:"Amplitude Controller Gain Get.vi"() -> ()  [unwired: 11 in, 5 out]
  n367 = call <userlib>:"Phase Controller Gain Get.vi"() -> ()  [unwired: 11 in, 5 out]
  n368 = call <userlib>:"FrequencyShift Get.vi"() -> ()  [unwired: 9 in, 3 out]
  n369 = call <userlib>:"PhaseSweep Start.vi"() -> ()  [unwired: 8 in, 4 out]
  n370 = call <userlib>:"FrqExc overwrite Get.vi"() -> ()  [unwired: 8 in, 4 out]
  n371 = call <userlib>:"Input Range Set.vi"() -> ()  [unwired: 10 in, 2 out]
  n372 = call <userlib>:"Amplitude Controller Gain Set.vi"() -> ()  [unwired: 10 in, 2 out]
  n373 = call <userlib>:"Phase Controller Gain Set.vi"() -> ()  [unwired: 10 in, 2 out]
  n374 = call <userlib>:"FrequencyShift Set.vi"() -> ()  [unwired: 10 in, 2 out]
  n375 = call <userlib>:"Prog Interface - OpenAppRef.vi"() -> ()  [unwired: 6 in, 2 out]
  n376 = call <userlib>:"TCP Receiver RT Oversampling Set.vi"() -> ()  [unwired: 10 in, 2 out]
  n377 = call <userlib>:"Load Settings File.vi"() -> ()  [unwired: 10 in, 2 out]
  n378 = call "Ms to Wait with error cluster.vi"() -> ()  [unwired: 6 in, 2 out]
  n379 = call <userlib>:"GenericSweep GetSweepSignal List.vi"() -> ()  [unwired: 9 in, 3 out]
  n380 = call <userlib>:"GenericSweep GetChannelsToRecord.vi"() -> ()  [unwired: 8 in, 4 out]
  n381 = call "Binary_SpectroscopyFile-Open.vi"() -> ()  [unwired: 7 in, 5 out]
  n382 = call <userlib>:"Create Header for BinaryFile.vi"() -> ()  [unwired: 11 in, 1 out]
  n383 = call "Load sxm File.vi"() -> ()  [unwired: 6 in, 6 out]
  n384 = call "Load dat File.vi"() -> ()  [unwired: 8 in, 4 out]
  n385 = call <userlib>:"Scan Action.vi"() -> ()  [unwired: 9 in, 2 out]
  n386 = call <userlib>:"Scan SetProperties.vi"() -> ()  [unwired: 14 in, 2 out]
  n387 = call <userlib>:"FolMe Speed Set.vi"() -> ()  [unwired: 8 in, 2 out]
  n388 = call <userlib>:"XY-Pos Set.vi"() -> ()  [unwired: 8 in, 2 out]
  n389 = call <userlib>:"Start Grid Experiment.vi"() -> ()  [unwired: 18 in, 2 out]
  n390 = call <userlib>:"Line Draw.vi"() -> ()  [unwired: 14 in, 2 out]
  n391 = call "Load nsp File.vi"() -> ()  [unwired: 6 in, 6 out]
  n392 = call <userlib>:"Point Draw.vi"() -> ()  [unwired: 14 in, 2 out]
  n393 = call-poly <userlib>:"Grid Pattern Get.vi"() -> ()  [unwired: 11 in, 9 out]
  n394 = call <userlib>:"FrqExc overwrite Set v3.vi"() -> ()  [unwired: 10 in, 2 out]
  n395 = call <userlib>:"Frequency Shift AutoCenter.vi"() -> ()  [unwired: 10 in, 2 out]
  n396 = call <userlib>:"Get Session Path.vi"() -> ()  [unwired: 9 in, 3 out]
  n397 = call <userlib>:"Set Session Path.vi"() -> ()  [unwired: 10 in, 2 out]
  n398 = call <userlib>:"TCP Receiver RT Oversampling Get.vi"() -> ()  [unwired: 9 in, 3 out]
  n399 = call <userlib>:"Save Settings File.vi"() -> ()  [unwired: 10 in, 2 out]
  n400 = call <userlib>:"Split Signal to Name and Unit.vi"() -> ()  [unwired: 6 in, 2 out]
  n401 = call "Binary_SpectroscopyFile-ReadData.vi"() -> ()  [unwired: 8 in, 4 out]
  n402 = call <userlib>:"Write Header to BinaryFile [ with Save dialog].vi"() -> ()  [unwired: 8 in, 4 out]
  n403 = call "Save sxm File.vi"() -> ()  [unwired: 9 in, 3 out]
  n404 = call <userlib>:"Save dat File.vi"() -> ()  [unwired: 12 in, 4 out]
  n405 = call <userlib>:"Scan WaitEOS.vi"() -> ()  [unwired: 7 in, 4 out]
  n406 = call <userlib>:"Scan GetProperties.vi"() -> ()  [unwired: 8 in, 8 out]
  n407 = call <instrlib>:"FolMe Speed Get.vi"() -> ()  [unwired: 6 in, 4 out]
  n408 = call <userlib>:"XY-Pos Set - Fast.vi"() -> ()  [unwired: 9 in, 2 out]
  n409 = call <userlib>:"Grid Experiment Status Get.vi"() -> ()  [unwired: 9 in, 3 out]
  n410 = call <userlib>:"Lines Draw.vi"() -> ()  [unwired: 14 in, 2 out]
  n411 = call <userlib>:"Points Draw.vi"() -> ()  [unwired: 14 in, 2 out]
  n412 = call <userlib>:"GenericSweep GetSweepSignal.vi"() -> ()  [unwired: 8 in, 4 out]
  n413 = call <userlib>:"GenericSweep SetChannelsToRecord.vi"() -> ()  [unwired: 10 in, 2 out]
  n414 = call <userlib>:"Add external signal on_off Get.vi"() -> ()  [unwired: 9 in, 3 out]
  n415 = call <userlib>:"Output (Exc) on_off Get.vi"() -> ()  [unwired: 9 in, 3 out]
  n416 = call <userlib>:"TCP Receiver Animations Period  Get.vi"() -> ()  [unwired: 9 in, 3 out]
  n417 = call <userlib>:"TCP Receiver Animations Period Set.vi"() -> ()  [unwired: 10 in, 2 out]
  n418 = call <userlib>:"Filter & Differentiation.vi"() -> ()  [unwired: 9 in, 3 out]
  n419 = call <userlib>:"Load Layout File.vi"() -> ()  [unwired: 10 in, 2 out]
  n420 = call <userlib>:"Append Unit to Signal Name.vi"() -> ()  [unwired: 7 in, 1 out]
  n421 = call "Binary_SpectroscopyFile-Close.vi"() -> ()  [unwired: 11 in, 1 out]
  n422 = call "Save dat File (Core).vi"() -> ()  [unwired: 14 in, 2 out]
  n423 = call <userlib>:"Scan Grab Frame Data.vi"() -> ()  [unwired: 11 in, 5 out]
  n424 = call <userlib>:"ScanBuffer Set.vi"() -> ()  [unwired: 14 in, 2 out]
  n425 = call <userlib>:"FolMe Oversampling Set.vi"() -> ()  [unwired: 8 in, 2 out]
  n426 = call <userlib>:"XY-Pos Get.vi"() -> ()  [unwired: 7 in, 4 out]
  n427 = call <userlib>:"Pause-Resume Grid Experiment.vi"() -> ()  [unwired: 18 in, 2 out]
  n428 = call <userlib>:"Line Erase.vi"() -> ()  [unwired: 14 in, 2 out]
  n429 = call <userlib>:"Point Erase.vi"() -> ()  [unwired: 14 in, 2 out]
  n430 = call <userlib>:"GenericSweep SetSweepSignal.vi"() -> ()  [unwired: 10 in, 2 out]
  n431 = call <userlib>:"GenericSweep Open.vi"() -> ()  [unwired: 14 in, 2 out]
  n432 = call <userlib>:"Add external signal on_off Set.vi"() -> ()  [unwired: 10 in, 2 out]
  n433 = call <userlib>:"Output (Exc) on_off Set.vi"() -> ()  [unwired: 10 in, 2 out]
  n434 = call-poly <userlib>:"Grid Pattern Set.vi"() -> ()  [unwired: 18 in, 2 out]
  n435 = call <userlib>:"Save Layout File.vi"() -> ()  [unwired: 10 in, 2 out]
  n436 = call <userlib>:"Lock Nanonis.vi"() -> ()  [unwired: 10 in, 2 out]
  n437 = call <userlib>:"UnLock Nanonis.vi"() -> ()  [unwired: 10 in, 2 out]
  n438 = call <userlib>:"Get All Parameters.vi"() -> ()  [unwired: 8 in, 4 out]
  n439 = call <userlib>:"Scan Status Get.vi"() -> ()  [unwired: 8 in, 3 out]
  n440 = call <userlib>:"ScanBuffer Get.vi"() -> ()  [unwired: 11 in, 5 out]
  n441 = call <userlib>:"FolMe Oversampling Get.vi"() -> ()  [unwired: 6 in, 4 out]
  n442 = call <userlib>:"FolMe Stop Movement.vi"() -> ()  [unwired: 8 in, 2 out]
  n443 = call <userlib>:"Stop Grid Experiment.vi"() -> ()  [unwired: 18 in, 2 out]
  n444 = call <userlib>:"Lines Get.vi"() -> ()  [unwired: 13 in, 3 out]
  n445 = call <userlib>:"Points Get.vi"() -> ()  [unwired: 13 in, 3 out]
  n446 = call <userlib>:"GenericSweep SetProperties.vi"() -> ()  [unwired: 14 in, 2 out]
  n447 = call <userlib>:"GenericSweep GetProperties.vi"() -> ()  [unwired: 9 in, 7 out]
  n448 = call <userlib>:"Global Counter Evaluate.vi"() -> ()  [unwired: 8 in, 4 out]
  n449 = call <userlib>:"Global Counter Get.vi"() -> ()  [unwired: 8 in, 4 out]
  n450 = call <userlib>:"Global Counter Set.vi"() -> ()  [unwired: 10 in, 2 out]
  n451 = call <userlib>:"SignalAnalyzer FFT GraphData Get.vi"() -> ()  [unwired: 9 in, 3 out]
  n452 = call <userlib>:"SignalAnalyzer Osci GraphData Get.vi"() -> ()  [unwired: 9 in, 3 out]
  n453 = call <userlib>:"SignalAnalyzer Open.vi"() -> ()  [unwired: 10 in, 2 out]
  n454 = call <userlib>:"SignalAnalyzer Osci GraphData Get.vi"() -> ()  [unwired: 9 in, 3 out]
  n455 = call <userlib>:"ZoomFFT Open.vi"() -> ()  [unwired: 10 in, 2 out]
  n456 = call <userlib>:"ZoomFFT GraphData Get.vi"() -> ()  [unwired: 9 in, 3 out]
  n457 = call <userlib>:"PLL Setup.vi"() -> ()  [unwired: 7 in, 5 out]
  n458 = call <userlib>:"TCP Receiver RT Frq Get.vi"() -> ()  [unwired: 9 in, 3 out]
  n459 = call <userlib>:"TCP Receiver RT Frq Set.vi"() -> ()  [unwired: 10 in, 2 out]
  n460 = call <userlib>:"ScanFrame Set.vi"() -> ()  [unwired: 14 in, 2 out]
  n461 = call <userlib>:"ScanFrame Get.vi"() -> ()  [unwired: 11 in, 5 out]
  n462 = call <userlib>:"FolMe Tip Recorder Data Save.vi"() -> ()  [unwired: 10 in, 2 out]
  n463 = call <userlib>:"FolMe Tip Recorder Data Get.vi"() -> ()  [unwired: 8 in, 4 out]
  n464 = call <userlib>:"Grid Experiments Get.vi"() -> ()  [unwired: 13 in, 7 out]
  n465 = call <userlib>:"Line ShowHide.vi"() -> ()  [unwired: 14 in, 2 out]
  n466 = call <userlib>:"Point ShowHide.vi"() -> ()  [unwired: 14 in, 2 out]
  n467 = call <userlib>:"GenericSweep SetLimits.vi"() -> ()  [unwired: 8 in, 2 out]
  n468 = call <userlib>:"GenericSweep GetLimits.vi"() -> ()  [unwired: 6 in, 4 out]
  n469 = call <userlib>:"SignalAnalyzer Channel Get.vi"() -> ()  [unwired: 7 in, 3 out]
  n470 = call <userlib>:"SignalAnalyzer Channel Set.vi"() -> ()  [unwired: 8 in, 2 out]
  n471 = call <userlib>:"SignalAnalyzer FFT GraphData Get.vi"() -> ()  [unwired: 9 in, 3 out]
  n472 = call <userlib>:"ZoomFFT Channel Get.vi"() -> ()  [unwired: 7 in, 3 out]
  n473 = call <userlib>:"ZoomFFT Channel Set.vi"() -> ()  [unwired: 8 in, 2 out]
  n474 = call <userlib>:"Speed Set.vi"() -> ()  [unwired: 14 in, 2 out]
  n475 = call <userlib>:"Speed Get.vi"() -> ()  [unwired: 10 in, 6 out]
  n476 = call <userlib>:"FolMe Tip Recorder Open.vi"() -> ()  [unwired: 8 in, 2 out]
  n477 = call <userlib>:"FolMe Tip Recorder Buffer Clear.vi"() -> ()  [unwired: 8 in, 2 out]
  n478 = call <userlib>:"Grid Experiment Set.vi"() -> ()  [unwired: 18 in, 2 out]
  n479 = call <userlib>:"GenericSweep Start.vi"() -> ()  [unwired: 12 in, 4 out]
  n480 = call <userlib>:"GenericSweep Stop.vi"() -> ()  [unwired: 14 in, 2 out]
  n481 = call <userlib>:"SignalAnalyzer Osci Trigger Properties Get.vi"() -> ()  [unwired: 6 in, 6 out]
  n482 = call <userlib>:"SignalAnalyzer Osci Trigger Properties Set.vi"() -> ()  [unwired: 10 in, 2 out]
  n483 = call <userlib>:"SignalAnalyzer Osci Trigger Auto.vi"() -> ()  [unwired: 10 in, 2 out]
  n484 = call <userlib>:"SignalAnalyzer FFT Averaging Restart.vi"() -> ()  [unwired: 10 in, 2 out]
  n485 = call <userlib>:"ZoomFFT Properties Get.vi"() -> ()  [unwired: 6 in, 4 out]
  n486 = call <userlib>:"ZoomFFT Properties Set.vi"() -> ()  [unwired: 8 in, 2 out]
  n487 = call <userlib>:"FolMe Tip Recorder Buffersize Set.vi"() -> ()  [unwired: 8 in, 2 out]
  n488 = call <userlib>:"FolMe Tip Recorder Buffersize Get.vi"() -> ()  [unwired: 7 in, 3 out]
  n489 = call "ScanMonitor.PI.Multiple.Generate.vi"() -> ()  [unwired: 1 in]
  n490 = call <userlib>:"Open Grid Experiment.vi"() -> ()  [unwired: 18 in, 2 out]
  n491 = call "Test connection.vi"() -> ()  [unwired: 1 in]
  n492 = call "StoreSpecParms.vi"() -> ()  [unwired: 1 in]
  n493 = call "Switch Mode STM-AFM.vi"() -> ()  [unwired: 1 in]
  n494 = call "ScanMonitor.PI.Multiple.Generate.vi"() -> ()  [unwired: 1 in]
  n495 = call "READ ME - External VI.vi"() -> ()  [unwired: 1 in]
  n496 = call "Binary_SpectroscopyFile-Plot3D-Surface.vi"() -> ()  [unwired: 12 in]
  n497 = call <userlib>:"SignalAnalyzer FFT Properties Get.vi"() -> ()  [unwired: 6 in, 4 out]
  n498 = call <userlib>:"SignalAnalyzer FFT Properties Set.vi"() -> ()  [unwired: 8 in, 2 out]
  n499 = call <userlib>:"SignalAnalyzer Osci Trigger Rearm.vi"() -> ()  [unwired: 10 in, 2 out]
  n500 = call <userlib>:"ZoomFFT Averaging Restart.vi"() -> ()  [unwired: 10 in, 2 out]
  n501 = call <userlib>:"Digital Line - SetProperties.vi"() -> ()  [unwired: 9 in, 3 out]
  n502 = call <userlib>:"Digital Lines - Pulse.vi"() -> ()  [unwired: 13 in, 3 out]
  n503 = call "GenericSweep - Multiple sweeps.vi"() -> ()  [unwired: 1 in]
  n504 = call "MultiSegmentSpectroscopy.vi"() -> ()  [unwired: 1 in]
  n505 = call "Switch scanners.vi"() -> ()  [unwired: 1 in]
  n506 = call "ScanMonitor.PI.Template.vit"() -> ()  [unwired: 12 in]
  n507 = call "Grid Measurements Example - MultipleSpectro.vi"() -> ()  [unwired: 11 in, 1 out]
  n508 = call "Binary_SpectroscopyFile-Read&ProcessTemplate.vi"() -> ()  [unwired: 1 in]
  n509 = call <userlib>:"SignalAnalyzer Timebase Get.vi"() -> ()  [unwired: 7 in, 5 out]
  n510 = call <userlib>:"SignalAnalyzer Timebase Set.vi"() -> ()  [unwired: 10 in, 2 out]
  n511 = call <userlib>:"Digital Line - SetStatus.vi"() -> ()  [unwired: 9 in, 3 out]
  n512 = call <userlib>:"Digital Lines - Get TTL Voltages.vi"() -> ()  [unwired: 8 in, 4 out]
  n513 = call "Custom Z Sweep (pt by pt).vi"() -> ()  [unwired: 1 in]
  n514 = call "User scan tool box.vi"() -> ()  [unwired: 1 in]
  n515 = call "ncAFM Amplitude Calibration.vi"() -> ()  [unwired: 1 in]
  n516 = call "Grid Measurements Example - Topo & GridSpectr.vi"() -> ()  [unwired: 11 in, 1 out]
  n517 = call "Binary_SpectroscopyFile-ExportSlices.vi"() -> ()  [unwired: 1 in]
  n518 = call <userlib>:"Demodulator PhaseReference Get.vi"() -> ()  [unwired: 9 in, 3 out]
  n519 = call <userlib>:"Demodulator Filter Set.vi"() -> ()  [unwired: 10 in, 2 out]
  n520 = call <userlib>:"Demodulator Harmonic Get.vi"() -> ()  [unwired: 9 in, 3 out]
  n521 = call <userlib>:"Demodulator Input Get.vi"() -> ()  [unwired: 8 in, 4 out]
  n522 = call <userlib>:"FunGen Start.vi"() -> ()  [unwired: 10 in, 2 out]
  n523 = call <userlib>:"FunGen Status Get.vi"() -> ()  [unwired: 8 in, 4 out]
  n524 = call <userlib>:"FunGen 2Ch Start.vi"() -> ()  [unwired: 10 in, 2 out]
  n525 = call <userlib>:"FunGen 2Ch Ch1 Channel Get.vi"() -> ()  [unwired: 8 in, 4 out]
  n526 = call <userlib>:"FunGen 2Ch Ch1 Channel Set.vi"() -> ()  [unwired: 10 in, 2 out]
  n527 = call <userlib>:"FunGen 2Ch Ch2 Channel Get.vi"() -> ()  [unwired: 8 in, 4 out]
  n528 = call <userlib>:"FunGen 2Ch Ch2 Channel Set.vi"() -> ()  [unwired: 10 in, 2 out]
  n529 = call "Custom Bias Sweep (pt by pt).vi"() -> ()  [unwired: 1 in]
  n530 = call "Scans at different Bias.vi"() -> ()  [unwired: 1 in]
  n531 = call "Feenstra type spectroscopy.vi"() -> ()  [unwired: 1 in]
  n532 = call "History Chart 1-Channel.vi"() -> ()  [unwired: 1 in]
  n533 = call "Grid Measurements Example - Potential.vi"() -> ()  [unwired: 11 in, 1 out]
  n534 = call "Grid Measurements Example - ExtractPointSpectro.vi"() -> ()  [unwired: 9 in, 3 out]
  n535 = call <userlib>:"Demodulator PhaseReference Set.vi"() -> ()  [unwired: 10 in, 2 out]
  n536 = call <userlib>:"Demodulator Filter Get.vi"() -> ()  [unwired: 7 in, 5 out]
  n537 = call <userlib>:"Demodulator Harmonic Set.vi"() -> ()  [unwired: 10 in, 2 out]
  n538 = call <userlib>:"Demodulator Input Set.vi"() -> ()  [unwired: 10 in, 2 out]
  n539 = call <userlib>:"FunGen Stop.vi"() -> ()  [unwired: 10 in, 2 out]
  n540 = call <userlib>:"FunGen 2Ch Status Get.vi"() -> ()  [unwired: 8 in, 4 out]
  n541 = call <userlib>:"FunGen 2Ch Ch1 Properties Get.vi"() -> ()  [unwired: 5 in, 7 out]
  n542 = call <userlib>:"FunGen 2Ch Ch1 Properties Set.vi"() -> ()  [unwired: 10 in, 2 out]
  n543 = call <userlib>:"FunGen 2Ch Ch2 Properties Get.vi"() -> ()  [unwired: 5 in, 7 out]
  n544 = call <userlib>:"FunGen 2Ch Ch2 Properties Set.vi"() -> ()  [unwired: 10 in, 2 out]
  n545 = call "2D Sweep using GenSweeper.vi"() -> ()  [unwired: 1 in]
  n546 = call "Tip Cleaner.vi"() -> ()  [unwired: 1 in]
  n547 = call "BiasSpectroscopy.vi"() -> ()  [unwired: 1 in]
  n548 = call "Grid Measurements with VISA connection to user instrument.vi"() -> ()  [unwired: 11 in, 1 out]
  n549 = call <userlib>:"FunGen Properties Set.vi"() -> ()  [unwired: 10 in, 2 out]
  n550 = call <userlib>:"FunGen Properties Get.vi"() -> ()  [unwired: 6 in, 6 out]
  n551 = call <userlib>:"FunGen 2Ch Stop.vi"() -> ()  [unwired: 10 in, 2 out]
  n552 = call <userlib>:"FunGen 2Ch Ch1 Waveform Get.vi"() -> ()  [unwired: 9 in, 3 out]
  n553 = call <userlib>:"FunGen 2Ch Ch1 Waveform Set.vi"() -> ()  [unwired: 10 in, 2 out]
  n554 = call <userlib>:"FunGen 2Ch Ch2 Waveform Get.vi"() -> ()  [unwired: 9 in, 3 out]
  n555 = call <userlib>:"FunGen 2Ch Ch2 Waveform Set.vi"() -> ()  [unwired: 10 in, 2 out]
  n556 = call "Voltage pulses at various Z.vi"() -> ()  [unwired: 1 in]
  n557 = call "Tip Shaper.vi"() -> ()  [unwired: 1 in]
  n558 = call "Draw Pattern Layer.vi"() -> ()  [unwired: 1 in]
  n559 = call <userlib>:"Laser on_off Set.vi"() -> ()  [unwired: 10 in, 2 out]
  n560 = call <userlib>:"Laser Properties Set.vi"() -> ()  [unwired: 10 in, 2 out]
  n561 = call <userlib>:"BeamDeflection Horizontal Config Set.vi"() -> ()  [unwired: 18 in, 2 out]
  n562 = call <userlib>:"BeamDeflection Vertical Config Set.vi"() -> ()  [unwired: 18 in, 2 out]
  n563 = call <userlib>:"BeamDeflection Intensity Config Set.vi"() -> ()  [unwired: 18 in, 2 out]
  n564 = call <userlib>:"BeamDeflection AutoOffset.vi"() -> ()  [unwired: 8 in, 2 out]
  n565 = call <userlib>:"FunGen 2Ch Idle Value Get.vi"() -> ()  [unwired: 9 in, 3 out]
  n566 = call <userlib>:"FunGen 2Ch Ch1 OnOff Get.vi"() -> ()  [unwired: 9 in, 3 out]
  n567 = call <userlib>:"FunGen 2Ch Ch1 OnOff Set.vi"() -> ()  [unwired: 10 in, 2 out]
  n568 = call <userlib>:"FunGen 2Ch Ch2 OnOff Get.vi"() -> ()  [unwired: 9 in, 3 out]
  n569 = call <userlib>:"FunGen 2Ch Ch2 OnOff Set.vi"() -> ()  [unwired: 10 in, 2 out]
  n570 = call <userlib>:"FunGen Idle Value Set.vi"() -> ()  [unwired: 9 in, 2 out]
  n571 = call <userlib>:"FunGen Idle Value Get.vi"() -> ()  [unwired: 9 in, 3 out]
  n572 = call "Point Shoot Example - MultipleSpectro.vi"() -> ()  [unwired: 11 in, 1 out]
  n573 = call "Force-Distance curve with offset compensation.vi"() -> ()  [unwired: 1 in]
  n574 = call "Z drift - measure and compensate.vi"() -> ()  [unwired: 1 in]
  n575 = call "Draw Scan Frame Outline.vi"() -> ()  [unwired: 1 in]
  n576 = call <userlib>:"Laser on_off Get.vi"() -> ()  [unwired: 9 in, 3 out]
  n577 = call <userlib>:"Laser Properties Get.vi"() -> ()  [unwired: 9 in, 3 out]
  n578 = call <userlib>:"Laser Power Get.vi"() -> ()  [unwired: 9 in, 3 out]
  n579 = call <userlib>:"BeamDeflection Horizontal Config Get.vi"() -> ()  [unwired: 14 in, 6 out]
  n580 = call <userlib>:"BeamDeflection Vertical Config Get.vi"() -> ()  [unwired: 14 in, 6 out]
  n581 = call <userlib>:"BeamDeflection Intensity Config Get.vi"() -> ()  [unwired: 14 in, 6 out]
  n582 = call "MultiPass - Example-Callback-VI.vi"() -> ()  [unwired: 11 in, 1 out]
  n583 = call <userlib>:"FunGen 2Ch Idle Value Set.vi"() -> ()  [unwired: 9 in, 2 out]
  n584 = call "Auto-Approach.vi"() -> ()  [unwired: 1 in]
  n585 = call "Convert SXM to PNG.vi"() -> ()  [unwired: 1 in]
  n586 = call "Get XY points from image.vi"() -> ()  [unwired: 1 in]
